vi "SetDriveEncoderPositions.vi"(1 "DriveEncoderRight":i32, 2 "DriveEncoderLeft":i32) -> ()   [LabVIEW 2017]
uses:
  <vilib>/Rock Robotics/Network Tables/NT Write Number.vi
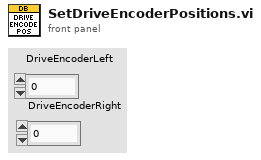
[diagram p1: front panel]
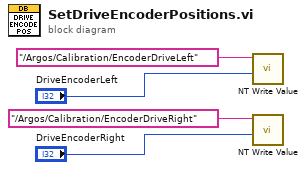
[diagram p0: block diagram]
diagram:
  n1 = call-poly <vilib>:"NT Write Value.vi"("Numeric"="DriveEncoderLeft", "Name"="/Argos/Calibration/EncoderDriveLeft") -> ()  [unwired: 9 in, 1 out]
  n2 = call-poly <vilib>:"NT Write Value.vi"("Numeric"="DriveEncoderRight", "Name"="/Argos/Calibration/EncoderDriveRight") -> ()  [unwired: 9 in, 1 out]
